vi "Get BLISS_PBQA and-or REJECTS.vi"(11 "BLISS Image Types":T1(ring)) -> (0 "Get PBQA":bool, 3 "Get Rejects":bool)   [LabVIEW 2020]
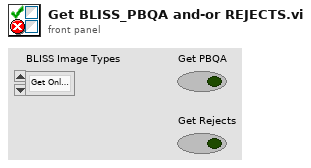
[diagram p1: front panel]
types:
  T1 = enum16{"Get Only Reject Images", "Get Only PBQA Images", "Get Both PBQA And Reject Images"}
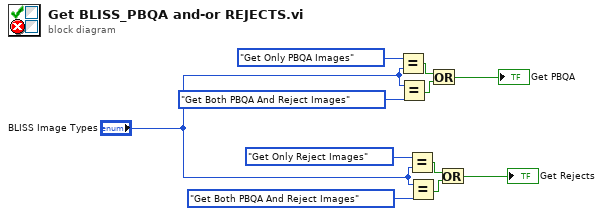
[diagram p0: block diagram]
diagram:
  n1 = Equal?(x=T1."Get Only PBQA Images" ("search criteria.BLISS Image Types"), y="BLISS Image Types") -> (x = y?=w3:bool)
  n2 = Equal?(x="BLISS Image Types", y=T1."Get Both PBQA And Reject Images" ("search criteria.BLISS Image Types")) -> (x = y?=w4:bool)
  n3 = Equal?(x=T1."Get Only Reject Images" ("search criteria.BLISS Image Types"), y="BLISS Image Types") -> (x = y?=w8:bool)
  n4 = Equal?(x="BLISS Image Types", y=T1."Get Both PBQA And Reject Images" ("search criteria.BLISS Image Types")) -> (x = y?=w7:bool)
  n5 = Or(x=w3, y=w4) -> (x .or. y?=→"Get PBQA":bool)
  n6 = Or(x=w8, y=w7) -> (x .or. y?=→"Get Rejects":bool)
